vi "PDLM_DecodeError.vi"(8 "error in (no error)":errorcluster, 10 "code":i32) -> (0 "error out":errorcluster, 2 "Error":string, 3 "return type":i32)   [LabVIEW 2019]
uses:
  <userlib>/TaikoLaser/PDLM_DllPath_global.vi
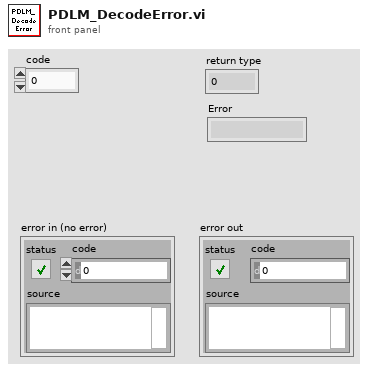
[diagram p1: front panel]
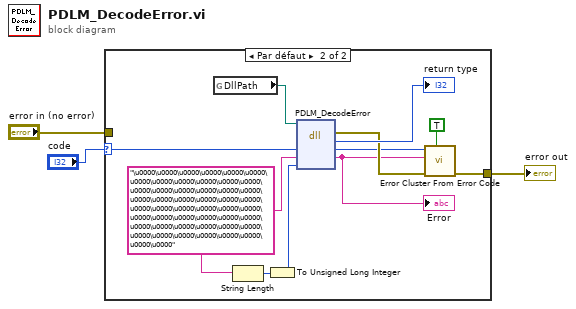
[diagram p0: block diagram]
diagram:
  n1 = case shown="Par défaut" "code" {
    selector: "code" -> [_ w10]
    tunnel: [w4 w12] -> w3
    tunnel: "error in (no error)" -> [w4 _]
    frame 0 {
    }
    frame Default {
      w9 = "\u0000\u0000\u0000\u0000\u0000\u0000\u0000\u0000\u0000\u0000\u0000\u0000\u0000\u0000\u0000\u0000\u0000\u0000\u0000\u0000\u0000\u0000\u0000\u0000\u0000\u0000\u0000\u0000\u0000\u0000\u0000\u0000\u0000\u0000\u0000\u0000\u0000\u0000\u0000\u0000\u0000\u0000\u0000\u0000\u0000\u0000\u0000\u0000\u0000\u0000" ("Version")
      n2 = global read "PDLM_DllPath_global.vi" "DllPath"() -> (w15:path)
      n3 = String Length(string=w9) -> (length=w8:i32)
      n4 = To Unsigned Long Integer(number=w8) -> (unsigned 32bit integer=w6:u32)
      n5 = dll-call lib="M:/_dev/progs/LabVIEW/_lib/PQ/Taiko/pdlm_lib.dll" fn="PDLM_DecodeError"(path in=w15, "Code"=w10, "Error"=w9, "BuffLen"=w6) -> (error out=w13:errorcluster, "return type"=→"return type":i32, "Code"=w7:i32, "Error"=w5:string)  [unwired: 3 in, 1 out]
      "Error" <- w5
      n6 = call <vilib>:"Error Cluster From Error Code.vi"("show call chain? (False)"=TRUE, "error in (no error)"=w13, "error message (\"\")"=w5, "error code (0)"=w7) -> ("error out"=w12:errorcluster)  [unwired: 5 in]
    }
  }
  "error out" <- w3
